vi "Read Lockin_Sweep.json.vi"(8 "error in (no error)":errorcluster, 10 "file (use dialog)":path, 11 "Transport in":refnum<class "SMO.Transport.lvclass">) -> (0 "error out":errorcluster, 2 "Configure Sweep":T1 {"Channels"."Channel" items=["AO1"=1, "AO2"=2]; "Channels"."Start" format="%#_6p"; "Channels"."End" format="%#_6p"}, 3 "Transport out":refnum<class "SMO.Transport.lvclass">)   [LabVIEW 2019, in "SMO.Transport.lvclass"]
uses:
  SMO.Transport.lvclass
  <vilib>/addons/_JKI.lib/Serialization/JSON/JKI JSON Serialization.lvlib
  <userlib>/LevyLab/Lockin-Multichannel/Lockin.DAQ/Typedefs/Sweep Configuration--Cluster.ctl
  <userlib>/LevyLab/Lockin-Multichannel/Lockin.DAQ/Typedefs/Sweep Pattern--Enum.ctl
  <userlib>/LevyLab/Lockin-Multichannel/Instrument.Lockinl.UI/Typedefs/Sweep Channel--Cluster.ctl
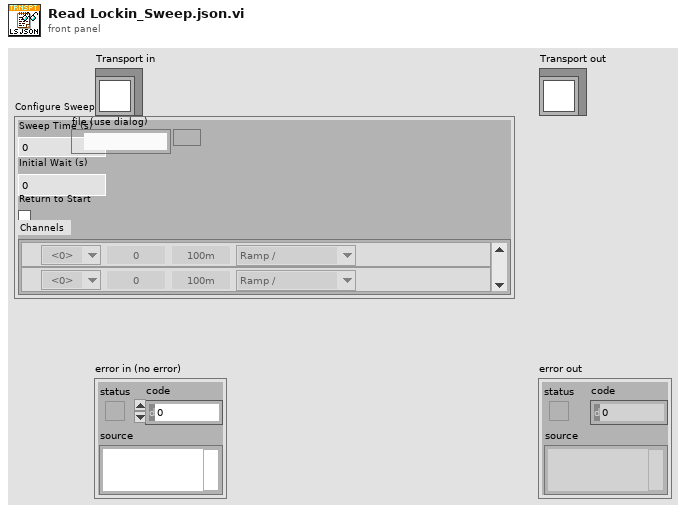
[diagram p1: front panel]
types:
  T1 = typedef "Lockin.DAQ.lvclass/Sweep Configuration--Cluster.ctl" = cluster{"Sweep Time (s)":dbl, "Initial Wait (s)":dbl, "Return to Start":bool, "Channels":T2[]}
  T2 = typedef "Instrument.Lockin.UI.lvclass/Sweep Channel--Cluster.ctl" = cluster{"End":dbl, "Start":dbl, "Channel":u16, "Pattern":T3}
  T3 = typedef "Lockin.DAQ.lvclass/Sweep Pattern--Enum.ctl" = enum16{"Ramp /", "Ramp /\\", "Smooth Ramp _/", "Smooth Ramp _/\\_", "Frequency"}
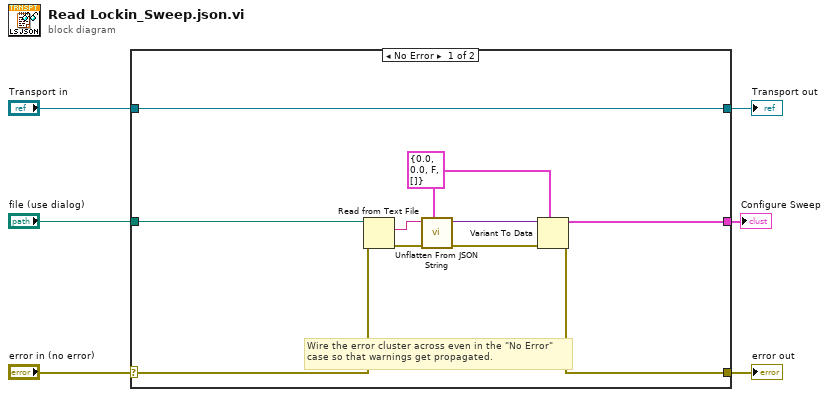
[diagram p0: block diagram]
diagram:
  n1 = case shown="No Error" "error in (no error)" {
    selector: "error in (no error)" -> [w8 w18]
    tunnel: [w7 w18] -> w5
    tunnel: [w16 w17] -> w3
    tunnel: "Transport in" -> [w16 w17]
    tunnel: [w10 _] -> w2
    tunnel: "file (use dialog)" -> [w9 _]
    frame No Error {
      w11 = T1 {"Sweep Time (s)"=0.0, "Initial Wait (s)"=0.0, "Return to Start"=FALSE, "Channels"=[]} ("Configure Sweep")
      # "Wire the error cluster across even in the \"No Error\"\ncase so that warnings get propagated."
      n2 = Read from Text File(file (use dialog)=w9, error in=w8) -> (text=w14:string, error out=w15:errorcluster)  [unwired: 2 in, 2 out]
      n3 = call <vilib>:"Unflatten From JSON String.vi"("Type and Defaults"=w11, "error in (no error)"=w15, "JSON String"=w14) -> ("error out"=w13:errorcluster, "Variant"=w12:variant)  [unwired: 7 in]
      n4 = Variant To Data(error in=w13, type=w11, Variant=w12) -> (data=w10:T1, error out=w7:errorcluster)
    }
    frame Error {
    }
  }
  "error out" <- w5
  "Transport out" <- w3
  "Configure Sweep" <- w2
